vi "Main.vi"() -> ()   [LabVIEW 2015, in "Serializer.lvlib"]
doc: "This template is based from the Queued Message Handler design pattern and the Queued Message Handler Project Template that ships with LabVIEW 2014.\n\nThe main difference is that the Queue is private to this module and communication between modules is done via Broadcast and Requests events.\n\nRequests events are wrapped via public API methods and are handled in the Event handler loop in this VI.\nAny module can register for Broadcast events sent by this module.\n\nThe Event Handling Loop generates messages based on user interface actions.\n\nThe Message Handling Loop processes messages generated by the Event Handling Loop, or by other messages. The messages are string values, so new messages can be added easily to the Message Cases case structure in the Message Handling Loop. Each message cluster can also provide an optional value for Message Data, which is a variant that can be converted to whatever message-specific data is required.\n_____\nBased on Delacor QMH Project Template 3.1.0.34."
uses:
  Serializer.lvlib
  <vilib>/Delacor/Delacor QMH/Libraries/Cloneable Module Admin_class/Delacor_lib_QMH_Cloneable Module Admin.lvclass
  Module Data--cluster.ctl
  OOP/Serial/Base/Serial.lvclass
  <vilib>/Delacor/Delacor QMH/Libraries/Cloneable Module Admin_class/Delacor_lib_QMH_Cloneable Module Admin.lvclass/Delacor_lib_QMH_Cloneable Module Admin.ctl
  Stop Argument--cluster.ctl
  <vilib>/Delacor/Delacor QMH/Libraries/Module Admin_class/Delacor_lib_QMH_Module Admin.lvclass/Delacor_lib_QMH_Module Admin.ctl
  Send Argument--cluster.ctl
  config Argument--cluster.ctl
  Open Argument--cluster.ctl
  close Argument--cluster.ctl
  PollRX Argument--cluster.ctl
  <vilib>/Utility/miscctls.llb/LVPointTypeDef.ctl
  <vilib>/Delacor/Delacor QMH/Libraries/Cloneable Module Admin_class/Delacor_lib_QMH_Get Module ID.vi
  <vilib>/Delacor/Delacor QMH/Libraries/Module Admin_class/Delacor_lib_QMH_Get External Launch.vi
  <vilib>/Delacor/Delacor QMH/Libraries/Message Queue_class/Delacor_lib_QMH_Enqueue Message (Single).vi
  <vilib>/Utility/error.llb/Error Cluster From Error Code.vi
  <vilib>/ErrorRing/Error Ring.xnode
  <vilib>/Delacor/Delacor QMH/Libraries/Message Queue_class/Delacor_lib_QMH_Message Queue.lvclass
  Clone Registration/Clone Registration.lvlib
panel:
  in  "Simulate MHL Error":bool
  in  "Simulate EHL Error":bool
  out "error out":errorcluster
  in  "Module Admin":refnum<class "Delacor_lib_QMH_Cloneable Module Admin.lvclass">
  out "Status":string
  # "Other QMH Modules communicate with this Module via its Public API (wrappers for its Request Events).\n\nThis Module communicates with other Modules via its Broadcast Events.\nAny module that wants to get these messages, just registers for this module's Broadcast events."
  # "This template is for the Delacor Modified Queued Message Handler design pattern.\n\nSee the block diagram for more information on how to use this template."
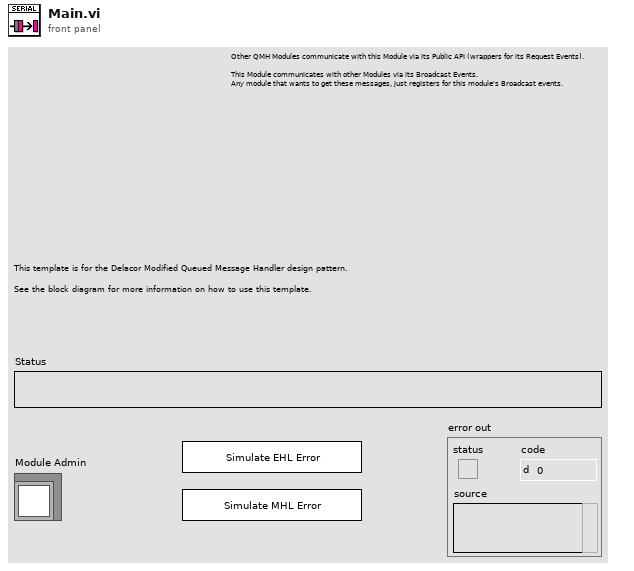
[diagram p1: front panel]
types:
  T1 = typedef "Serializer.lvlib/Request Events--cluster.ctl" = cluster{"Stop Module":refnum<user-event>, "Show Panel":refnum<user-event>, "Hide Panel":refnum<user-event>, "Show Diagram":refnum<user-event>, "Get Module Execution Status":refnum<user-event>, "Send":refnum<user-event>, "config":refnum<user-event>, "Open":refnum<user-event>, "close":refnum<user-event>, "PollRX":refnum<user-event>}
  T2 = typedef "Serializer.lvlib/Module Data--cluster.ctl" = cluster{"Status":string, "Serial.lvclass":refnum<class "Serial.lvclass">}
  T3 = typedef "Serializer.lvlib/Stop Argument--cluster.ctl" = cluster{"Origin":string, "Module ID":i32, "Exit via Stop Module Req?":bool, "Wait for Module to stop?":bool}
  T4 = typedef "Serializer.lvlib/Send Argument--cluster.ctl" = cluster{"Module ID":i32, "Bytes":u8[]}
  T5 = typedef "Serializer.lvlib/config Argument--cluster.ctl" = cluster{"Module ID":i32, "config":string}
  T6 = typedef "Serializer.lvlib/Open Argument--cluster.ctl" = cluster{"Module ID":i32, "Boolean":bool}
  T7 = typedef "Serializer.lvlib/close Argument--cluster.ctl" = cluster{"Module ID":i32, "Boolean":bool}
  T8 = typedef "Serializer.lvlib/PollRX Argument--cluster.ctl" = cluster{"Module ID":i32, "Boolean":bool}
  T9 = typedef "LVPointTypeDef.ctl" = cluster{"Horizontal":i16, "Vertical":i16}
  T10 = enum32{"Invalid", "Standard", "Closed", "Hidden", "Minimized", "Maximized"}
  T11 = enum32{"invalid lock state", "Not Locked", "Locked (No Password)", "Password-protected"}
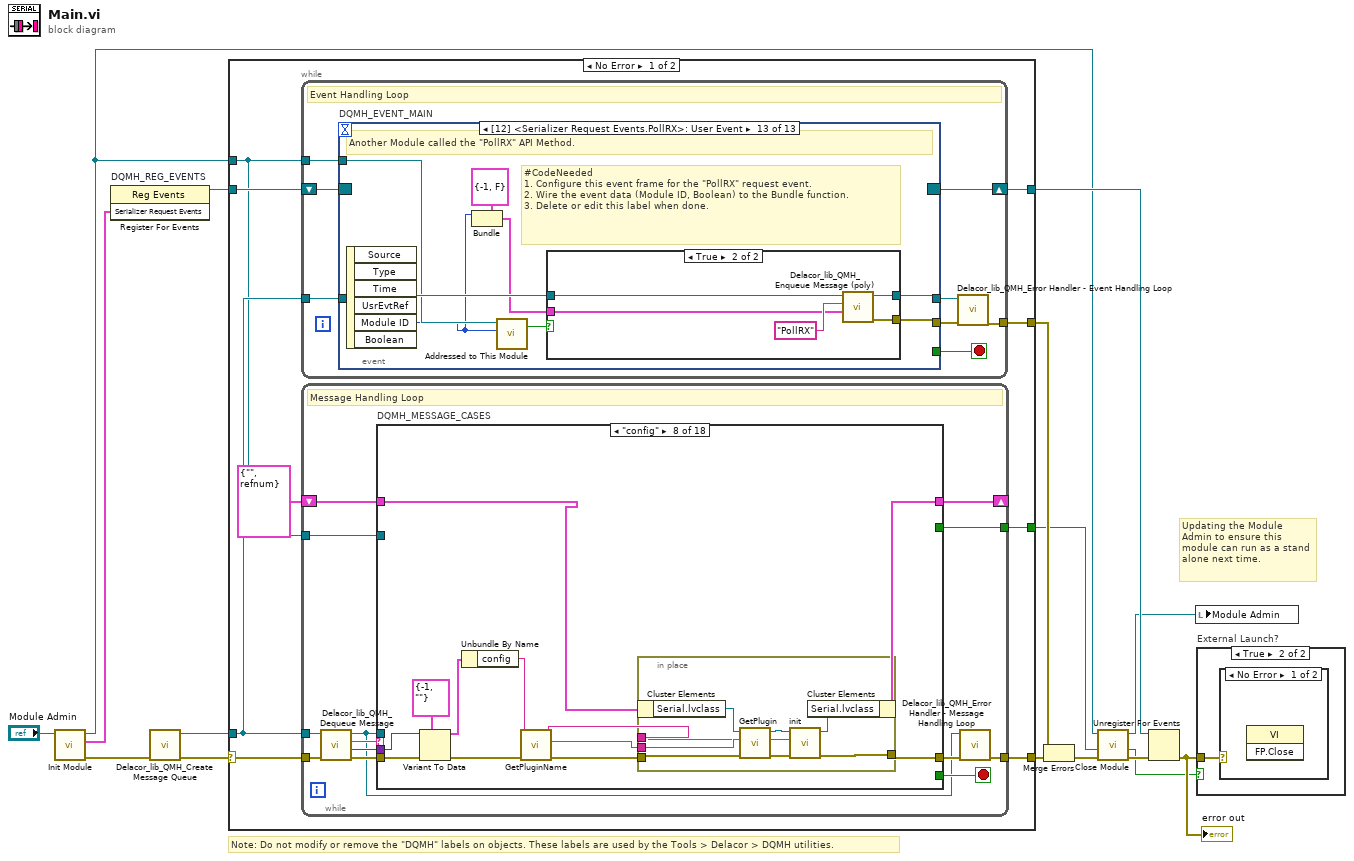
[diagram p0: block diagram]
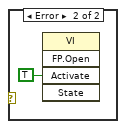
[diagram p3: hidden frame]
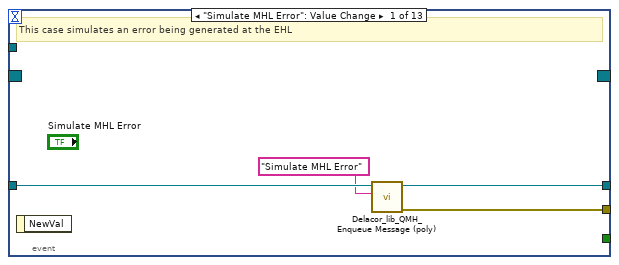
[diagram p4: hidden frame]
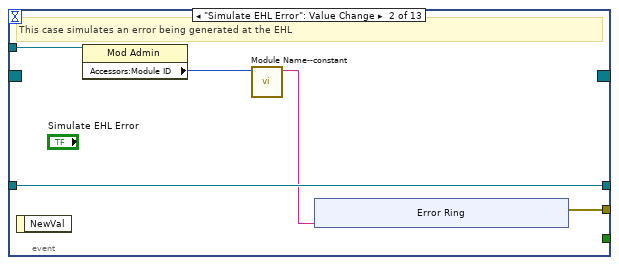
[diagram p5: hidden frame]
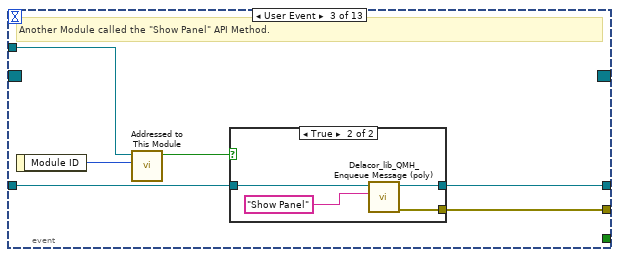
[diagram p6: hidden frame]
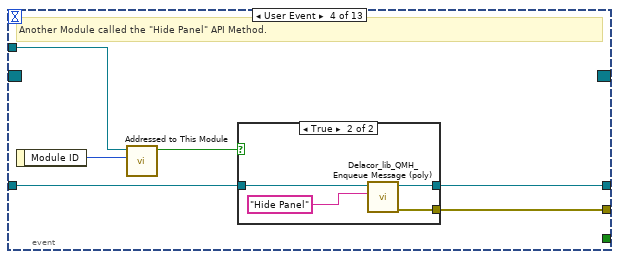
[diagram p8: hidden frame]
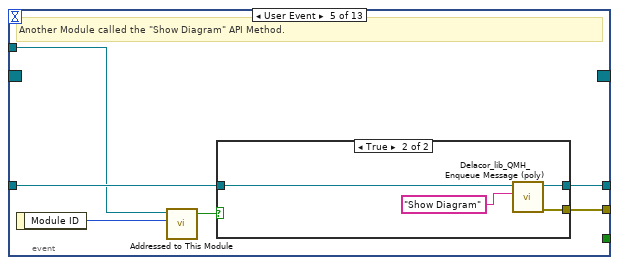
[diagram p10: hidden frame]
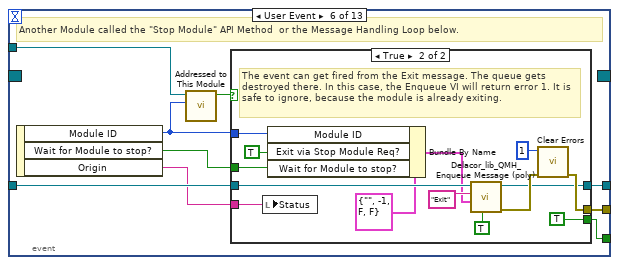
[diagram p12: hidden frame]
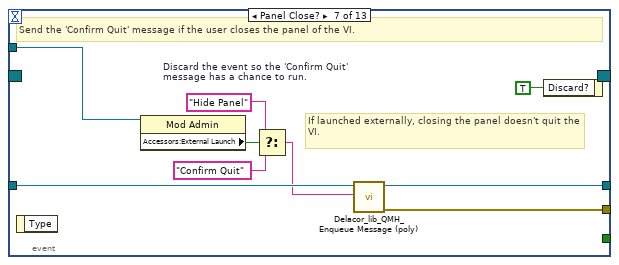
[diagram p14: hidden frame]
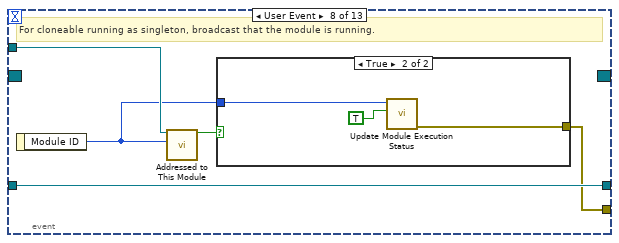
[diagram p15: hidden frame]
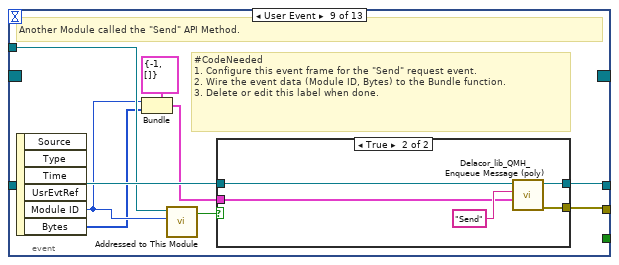
[diagram p17: hidden frame]
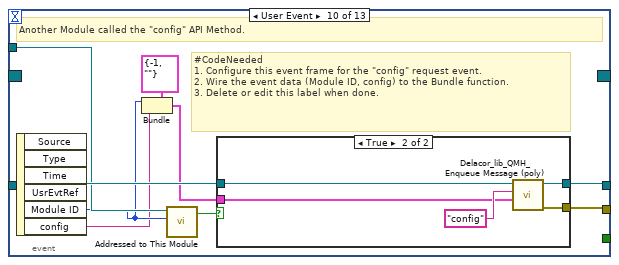
[diagram p19: hidden frame]
diagram:
  # "Note: Do not modify or remove the \"DQMH\" labels on objects. These labels are used by the Tools > Delacor > DQMH utilities."
  # "Updating the Module Admin to ensure this module can run as a stand alone next time."
  n1 = call "Init Module.vi"("Cloneable Module Admin in"="Module Admin") -> ("error out"=w13:errorcluster, "Serializer Request Events"=w10:T1, "Cloneable Module Admin out"=w6:refnum<class "Delacor_lib_QMH_Cloneable Module Admin.lvclass">)  [unwired: 8 in]
  n2 = register-events "DQMH_REG_EVENTS"(w10) -> (reference out=w11:refnum<event-registration>)  [unwired: 2 in, 1 out]
  n3 = call <vilib>:"Delacor_lib_QMH_Create Message Queue.vi"("error in (no error)"=w13) -> ("error out"=w1:errorcluster, "Message Queue out"=w9:refnum<class "Delacor_lib_QMH_Message Queue.lvclass">)  [unwired: 9 in]
  n4 = case shown="No Error" w1 {
    selector: w1 -> [w19 w447]
    tunnel: [w25 w447] -> w14
    tunnel: [w24 w448] -> w12
    tunnel: w11 -> [w22 w448]
    tunnel: w9 -> [w21 _]
    tunnel: [w20 _] -> w15
    tunnel: w6 -> [w18 w443]
    tunnel: [w17 _] -> w4
    frame No Error {
      n5 = while {
        tunnel: w21 -> [w33]
        shift-right: [w31] -> w24
        shift-left: w22 -> [w32]
        tunnel: [w27] -> w20
        tunnel: w18 -> [w26]
        stop <- w29 stop-if-true
        # "Event Handling Loop"
        n6 = event "DQMH_EVENT_MAIN" shown="[12] <Serializer Request Events.PollRX>: User Event" {
          selector: w32 -> [_ _ _ _ _ _ _ _ _ _ _ _ _]
          dyn-events: [_ _ _ _ _ _ _ _ _ _ _ _ _] -> w31
          timeout: _ -> [_ _ _ _ _ _ _ _ _ _ _ _ _]
          tunnel: [_ _ _ _ _ w86 _ _ _ _ _ _ _] -> w29
          tunnel: w33 -> [w37 w42 w55 w66 w77 w89 w114 w118 w132 w147 w161 w175 w189]
          tunnel: [w35 w41 w53 w64 w73 w91 w113 w117 w126 w141 w155 w169 w183] -> w30
          tunnel: [w36 w42 w54 w65 w76 w90 w112 w118 w131 w146 w160 w174 w188] -> w28
          tunnel: w26 -> [_ w40 w50 w61 w74 w88 w108 w119 w129 w144 w158 w172 w186]
          event "Simulate MHL Error": Value Change {
            # "This case simulates an error being generated at the EHL"
            n7 = event-data() -> ()  [unwired: 1 in, 1 out]
            n8 = call-poly <vilib>:"Delacor_lib_QMH_Enqueue Message (poly).vi"("Message"="Simulate MHL Error", "Message Queue in"=w37) -> ("error out"=w35:errorcluster, "Message Queue out"=w36:refnum<class "Delacor_lib_QMH_Message Queue.lvclass">)  [unwired: 8 in]
          }
          event "Simulate EHL Error": Value Change {
            # "This case simulates an error being generated at the EHL"
            n9 = event-data() -> ()  [unwired: 1 in, 1 out]
            n10 = property class="Mod Admin"(reference=w40) -> ("Accessors:Module ID"=w39:i32)  [unwired: 1 in, 2 out]
            n11 = call "Module Name--constant.vi"("Module ID"=w39) -> ("Module Name"=w38:string)  [unwired: 10 in]
            n12 = xnode "Error Ring"("parameter 0"=w38) -> ("error out"=w41:errorcluster)
          }
          event User Event {
            # "Another Module called the \"Show Panel\" API Method."
            n13 = event-data() -> ("Module ID"=w52:i32)  [unwired: 1 in]
            n14 = call "Addressed to This Module.vi"("Module ID from Argument"=w52, "Module Admin"=w50) -> ("Addressed to this instance?"=w51:bool)  [unwired: 8 in, 1 out]
            n15 = case shown="True" w51 {
              tunnel: w55 -> [w56 w60]
              tunnel: [w56 w59] -> w54
              tunnel: [_ w58] -> w53
              frame False {
              }
              frame True {
                n16 = call-poly <vilib>:"Delacor_lib_QMH_Enqueue Message (poly).vi"("Message"="Show Panel", "Message Queue in"=w60) -> ("error out"=w58:errorcluster, "Message Queue out"=w59:refnum<class "Delacor_lib_QMH_Message Queue.lvclass">)  [unwired: 8 in]
              }
            }
          }
          event User Event {
            # "Another Module called the \"Hide Panel\" API Method."
            n17 = event-data() -> ("Module ID"=w63:i32)  [unwired: 1 in]
            n18 = call "Addressed to This Module.vi"("Module ID from Argument"=w63, "Module Admin"=w61) -> ("Addressed to this instance?"=w62:bool)  [unwired: 8 in, 1 out]
            n19 = case shown="True" w62 {
              tunnel: w66 -> [w67 w71]
              tunnel: [w67 w70] -> w65
              tunnel: [_ w69] -> w64
              frame False {
              }
              frame True {
                n20 = call-poly <vilib>:"Delacor_lib_QMH_Enqueue Message (poly).vi"("Message"="Hide Panel", "Message Queue in"=w71) -> ("error out"=w69:errorcluster, "Message Queue out"=w70:refnum<class "Delacor_lib_QMH_Message Queue.lvclass">)  [unwired: 8 in]
              }
            }
          }
          event User Event {
            # "Another Module called the \"Show Diagram\" API Method."
            n21 = event-data() -> ("Module ID"=w72:i32)  [unwired: 1 in]
            n22 = call "Addressed to This Module.vi"("Module ID from Argument"=w72, "Module Admin"=w74) -> ("Addressed to this instance?"=w75:bool)  [unwired: 8 in, 1 out]
            n23 = case shown="True" w75 {
              tunnel: w77 -> [w78 w82]
              tunnel: [w78 w81] -> w76
              tunnel: [_ w79] -> w73
              frame False {
              }
              frame True {
                n24 = call-poly <vilib>:"Delacor_lib_QMH_Enqueue Message (poly).vi"("Message"="Show Diagram", "Message Queue in"=w82) -> ("error out"=w79:errorcluster, "Message Queue out"=w81:refnum<class "Delacor_lib_QMH_Message Queue.lvclass">)  [unwired: 8 in]
              }
            }
          }
          event User Event {
            # "Another Module called the \"Stop Module\" API Method  or the Message Handling Loop below."
            n25 = event-data() -> ("Module ID"=w84:i32, "Wait for Module to stop?"=w85:bool, "Origin"=w83:string)  [unwired: 1 in]
            n26 = call "Addressed to This Module.vi"("Module ID from Argument"=w84, "Module Admin"=w88) -> ("Addressed to this instance?"=w87:bool)  [unwired: 8 in, 1 out]
            n27 = case shown="True" w87 {
              tunnel: [_ w102] -> w91
              tunnel: [w92 w101] -> w90
              tunnel: w89 -> [w92 w100]
              tunnel: [_ TRUE] -> w86
              tunnel: w85 -> [_ w95]
              tunnel: w84 -> [_ w97]
              tunnel: w83 -> [_ w93]
              frame False {
              }
              frame True {
                # "The event can get fired from the Exit message. The queue gets destroyed there. In this case, the Enqueue VI will return error 1. It is safe to ignore, because the module is already exiting."
                n28 = local write "Status"(w93) -> ()
                n29 = Bundle By Name(cluster=T3 {"Origin"="", "Module ID"=-1, "Exit via Stop Module Req?"=FALSE, "Wait for Module to stop?"=FALSE} ("Stop Argument"), "Module ID"=w97, "Exit via Stop Module Req?"=TRUE, "Wait for Module to stop?"=w95) -> (w94:T3)
                n30 = call-poly <vilib>:"Delacor_lib_QMH_Enqueue Message (poly).vi"("Priority Message? (F)"=TRUE, "Message Data"=w94, "Message"="Exit", "Message Queue in"=w100) -> ("error out"=w105:errorcluster, "Message Queue out"=w101:refnum<class "Delacor_lib_QMH_Message Queue.lvclass">)  [unwired: 6 in]
                n31 = call <vilib>:"Clear Errors.vi"("error in (no error)"=w105, "specific error code to clear (0: all)"=1) -> ("error out"=w102:errorcluster)  [unwired: 4 in, 1 out]
              }
            }
          }
          event Panel Close? {
            w115 = TRUE  # Discard the event so the 'Confirm Quit' message has a chance to run.
            # "If launched externally, closing the panel doesn't quit the VI."
            # "Send the 'Confirm Quit' message if the user closes the panel of the VI."
            n32 = event-data() -> ()  [unwired: 1 in, 1 out]
            n33 = property class="Mod Admin"(reference=w108) -> ("Accessors:External Launch"=w107:bool)  [unwired: 1 in, 2 out]
            n34 = Select(t="Hide Panel" ("Message"), s=w107, f="Confirm Quit" ("Message")) -> (s? t:f=w109:string)
            n35 = call-poly <vilib>:"Delacor_lib_QMH_Enqueue Message (poly).vi"("Message"=w109, "Message Queue in"=w114) -> ("error out"=w113:errorcluster, "Message Queue out"=w112:refnum<class "Delacor_lib_QMH_Message Queue.lvclass">)  [unwired: 8 in]
            n36 = event-data("Discard?"=w115) -> ()  [unwired: 1 in, 1 out]
          }
          event User Event {
            # "For cloneable running as singleton, broadcast that the module is running."
            n37 = event-data() -> ("Module ID"=w116:i32)  [unwired: 1 in]
            n38 = call "Addressed to This Module.vi"("Module ID from Argument"=w116, "Module Admin"=w119) -> ("Addressed to this instance?"=w120:bool)  [unwired: 8 in, 1 out]
            n39 = case shown="True" w120 {
              tunnel: [_ w123] -> w117
              tunnel: w116 -> [_ w122]
              frame False {
              }
              frame True {
                n40 = call "Update Module Execution Status.vi"("Running?"=TRUE, "Module ID"=w122) -> ("error out"=w123:errorcluster)  [unwired: 9 in]
              }
            }
          }
          event User Event {
            # "#CodeNeeded\n1. Configure this event frame for the \"Send\" request event.\n2. Wire the event data (Module ID, Bytes) to the Bundle function.\n3. Delete or edit this label when done."
            # "Another Module called the \"Send\" API Method."
            n41 = event-data() -> ("Module ID"=w125:i32, "Bytes"=w124:u8[])  [unwired: 1 in, 4 out]
            n42 = Bundle(cluster=T4 {"Module ID"=-1, "Bytes"=[]} ("Send Argument"), "Module ID"=w125, "Bytes"=w124) -> (w127:T4)
            n43 = call "Addressed to This Module.vi"("Module ID from Argument"=w125, "Module Admin"=w129) -> ("Addressed to this instance?"=w130:bool)  [unwired: 8 in, 1 out]
            n44 = case shown="True" w130 {
              tunnel: w132 -> [w133 w138]
              tunnel: [w133 w137] -> w131
              tunnel: w127 -> [_ w135]
              tunnel: [_ w134] -> w126
              frame False {
              }
              frame True {
                n45 = call-poly <vilib>:"Delacor_lib_QMH_Enqueue Message (poly).vi"("Message Data"=w135, "Message"="Send", "Message Queue in"=w138) -> ("error out"=w134:errorcluster, "Message Queue out"=w137:refnum<class "Delacor_lib_QMH_Message Queue.lvclass">)  [unwired: 7 in]
              }
            }
          }
          event User Event {
            # "#CodeNeeded\n1. Configure this event frame for the \"config\" request event.\n2. Wire the event data (Module ID, config) to the Bundle function.\n3. Delete or edit this label when done."
            # "Another Module called the \"config\" API Method."
            n46 = event-data() -> ("Module ID"=w140:i32, "config"=w139:string)  [unwired: 1 in, 4 out]
            n47 = Bundle(cluster=T5 {"Module ID"=-1, "config"=""} ("config Argument"), "Module ID"=w140, "config"=w139) -> (w142:T5)
            n48 = call "Addressed to This Module.vi"("Module ID from Argument"=w140, "Module Admin"=w144) -> ("Addressed to this instance?"=w145:bool)  [unwired: 8 in, 1 out]
            n49 = case shown="True" w145 {
              tunnel: w147 -> [w148 w153]
              tunnel: [w148 w152] -> w146
              tunnel: w142 -> [_ w150]
              tunnel: [_ w149] -> w141
              frame False {
              }
              frame True {
                n50 = call-poly <vilib>:"Delacor_lib_QMH_Enqueue Message (poly).vi"("Message Data"=w150, "Message"="config", "Message Queue in"=w153) -> ("error out"=w149:errorcluster, "Message Queue out"=w152:refnum<class "Delacor_lib_QMH_Message Queue.lvclass">)  [unwired: 7 in]
              }
            }
          }
          event User Event {
            # "#CodeNeeded\n1. Configure this event frame for the \"Open\" request event.\n2. Wire the event data (Module ID, Boolean) to the Bundle function.\n3. Delete or edit this label when done."
            # "Another Module called the \"Open\" API Method."
            n51 = event-data() -> ("Module ID"=w154:i32)  [unwired: 1 in, 5 out]
            n52 = Bundle(cluster=T6 {"Module ID"=-1, "Boolean"=FALSE} ("Open Argument"), "Module ID"=w154) -> (w156:T6)  [unwired: 1 in]
            n53 = call "Addressed to This Module.vi"("Module ID from Argument"=w154, "Module Admin"=w158) -> ("Addressed to this instance?"=w159:bool)  [unwired: 8 in, 1 out]
            n54 = case shown="True" w159 {
              tunnel: w161 -> [w162 w167]
              tunnel: [w162 w166] -> w160
              tunnel: w156 -> [_ w164]
              tunnel: [_ w163] -> w155
              frame False {
              }
              frame True {
                n55 = call-poly <vilib>:"Delacor_lib_QMH_Enqueue Message (poly).vi"("Message Data"=w164, "Message"="Open", "Message Queue in"=w167) -> ("error out"=w163:errorcluster, "Message Queue out"=w166:refnum<class "Delacor_lib_QMH_Message Queue.lvclass">)  [unwired: 7 in]
              }
            }
          }
          event User Event {
            # "#CodeNeeded\n1. Configure this event frame for the \"close\" request event.\n2. Wire the event data (Module ID, Boolean) to the Bundle function.\n3. Delete or edit this label when done."
            # "Another Module called the \"close\" API Method."
            n56 = event-data() -> ("Module ID"=w168:i32)  [unwired: 1 in, 5 out]
            n57 = Bundle(cluster=T7 {"Module ID"=-1, "Boolean"=FALSE} ("close Argument"), "Module ID"=w168) -> (w170:T7)  [unwired: 1 in]
            n58 = call "Addressed to This Module.vi"("Module ID from Argument"=w168, "Module Admin"=w172) -> ("Addressed to this instance?"=w173:bool)  [unwired: 8 in, 1 out]
            n59 = case shown="True" w173 {
              tunnel: w175 -> [w176 w181]
              tunnel: [w176 w180] -> w174
              tunnel: w170 -> [_ w178]
              tunnel: [_ w177] -> w169
              frame False {
              }
              frame True {
                n60 = call-poly <vilib>:"Delacor_lib_QMH_Enqueue Message (poly).vi"("Message Data"=w178, "Message"="close", "Message Queue in"=w181) -> ("error out"=w177:errorcluster, "Message Queue out"=w180:refnum<class "Delacor_lib_QMH_Message Queue.lvclass">)  [unwired: 7 in]
              }
            }
          }
          event User Event {
            # "#CodeNeeded\n1. Configure this event frame for the \"PollRX\" request event.\n2. Wire the event data (Module ID, Boolean) to the Bundle function.\n3. Delete or edit this label when done."
            # "Another Module called the \"PollRX\" API Method."
            n61 = event-data() -> ("Module ID"=w182:i32)  [unwired: 1 in, 5 out]
            n62 = Bundle(cluster=T8 {"Module ID"=-1, "Boolean"=FALSE} ("PollRX Argument"), "Module ID"=w182) -> (w184:T8)  [unwired: 1 in]
            n63 = call "Addressed to This Module.vi"("Module ID from Argument"=w182, "Module Admin"=w186) -> ("Addressed to this instance?"=w187:bool)  [unwired: 8 in, 1 out]
            n64 = case shown="True" w187 {
              tunnel: w189 -> [w190 w195]
              tunnel: [w190 w194] -> w188
              tunnel: w184 -> [_ w192]
              tunnel: [_ w191] -> w183
              frame False {
              }
              frame True {
                n65 = call-poly <vilib>:"Delacor_lib_QMH_Enqueue Message (poly).vi"("Message Data"=w192, "Message"="PollRX", "Message Queue in"=w195) -> ("error out"=w191:errorcluster, "Message Queue out"=w194:refnum<class "Delacor_lib_QMH_Message Queue.lvclass">)  [unwired: 7 in]
              }
            }
          }
        }
        n66 = call-dynamic "Delacor_lib_QMH_Error Handler - Event Handling Loop.vi"("error in (no error)"=w30, "Message Queue in"=w28) -> ("dup error in"=w27:errorcluster)  [unwired: 8 in, 1 out]
      }
      n67 = while {
        tunnel: w21 -> [w200]
        shift-right: [w206] -> _
        shift-left: T2 {"Status"="", "Serial.lvclass"=refnum} ("Data Cluster") -> [w207]
        tunnel: w19 -> [w204]
        tunnel: [w198] -> w25
        tunnel: w18 -> [w197]
        tunnel: [w196] -> w17
        stop <- w205 stop-if-true
        # "Message Handling Loop"
        n68 = call-dynamic "Delacor_lib_QMH_Dequeue Message.vi"("error in (no error)"=w204, "Message Queue in"=w200) -> ("error out"=w203:errorcluster, "Message Data"=w201:variant, "Message"=w202:string, "Message Queue out"=w199:refnum<class "Delacor_lib_QMH_Message Queue.lvclass">)  [unwired: 6 in]
        n69 = case "DQMH_MESSAGE_CASES" shown="\"config\"" w202 {
          selector: w202 -> [_ _ _ _ _ _ _ _ _ _ _ _ _ _ _ _ _ w430]
          tunnel: w199 -> [_ _ _ _ _ _ _ _ _ _ _ _ _ w374 _ w407 w424 _]
          tunnel: w203 -> [w221 w237 w245 w251 w254 w275 w286 w298 w315 w328 w346 w369 w372 w383 w396 w406 w426 _]
          tunnel: [w214 w238 w245 w251 w253 w273 w276 w293 w310 w322 w337 w367 w370 w373 w394 w405 w420 w431] -> w208
          tunnel: w207 -> [w220 w239 w244 w250 w255 w274 w281 w288 w309 w325 w342 w368 w371 w382 w395 w410 w423 w432]
          tunnel: [w219 w239 w244 w250 w255 w274 w280 w294 w308 w324 w341 w368 w371 w382 w395 w410 w423 w432] -> w206
          tunnel: [_ _ _ _ _ _ _ _ _ _ _ _ _ _ _ _ w422 _] -> w205
          tunnel: w201 -> [_ w236 _ _ _ _ w285 w297 w314 w327 w345 _ _ w381 _ _ w416 _]
          tunnel: w197 -> [w211 w231 w242 w249 w252 _ _ _ _ _ _ _ _ w378 w391 _ w412 w428]
          tunnel: [_ _ _ _ _ _ _ _ _ _ _ _ _ _ _ _ w414 _] -> w196
          frame "Initialize" {
            w218 = "Initial Message" ("Initial Message")
            # "#CodeNeeded - Initialize the appearance of the front panel."
            # "#CodeNeeded - Initialize your state data here."
            # "Initialize - Any operation that needs to be done before the module can receive messages. Synchronize Caller Events.vi will inform Start Module.vi that the module has launched and is ready to receive messages. Module Did Init.vi will broadcast that the module initialized."
            n70 = call "Synchronize Caller Events.vi"("error in (no error)"=w221, "Module Admin"=w211) -> ("error out"=w215:errorcluster, "Module Admin out"=w210:refnum<class "Delacor_lib_QMH_Cloneable Module Admin.lvclass">)  [unwired: 8 in]
            n71 = property class="Mod Admin"(reference=w210) -> ("Accessors:Module ID"=w213:i32, "Accessors:External Launch"=w212:bool)  [unwired: 1 in, 2 out]
            n72 = call "Module Name--constant.vi"("Module ID"=w213) -> ("Module Name"=w225:string)  [unwired: 10 in]
            n73 = property class="VI"("Front Panel.Title"=w225) -> (reference out=w228:refnum<vi>, error out=w229:errorcluster)  [unwired: 2 in]
            n74 = Select(t=T10."Hidden" ("State"), s=w212, f=T10."Standard" ("State")) -> (s? t:f=w222:T10)
            n75 = invoke class="VI" method="FP.Open"(reference=w228, error in=w229, "State"=w222) -> (reference out=w227:refnum<vi>, error out=w226:errorcluster)  [unwired: 2 in, 3 out]
            n76 = call "Module Name--constant.vi"("Module ID"=w213) -> ("Module Name"=w216:string)  [unwired: 10 in]
            n77 = Bundle By Name(cluster=w220, "Status"=w218) -> (w219:T2)
            n78 = local write "Status"(w218) -> ()
            n79 = invoke class="VI" method="FP.Center"(reference=w227, error in=w226) -> ()  [unwired: 1 in, 3 out]
            n80 = property on="Pane" class="Pane"("Origin"=T9 {"Horizontal"=0, "Vertical"=0}) -> ()  [unwired: 2 in, 2 out]
            n81 = call "Module Did Init.vi"("error in (no error)"=w215, "Initialized?"=TRUE, "Origin"=w216, "Module ID"=w213) -> ("error out"=w214:errorcluster)  [unwired: 7 in]
          }
          frame "Update Display" {
            # "Broadcast updated status to any VI registered to listen to this module's broadcast events."
            # "Convert the message data to a string to display in the Status indicator."
            # "#CodeRecommended - If you wish to decouple the Message Handling Loop from your user interface, consider creating User Events (like the \"Stop\" event in this VI) to message the Event Handling Loop whenever the user interface needs updating."
            # "Update Display - Update user interface here."
            n82 = Variant To Data(error in=w237, type="", Variant=w236) -> (data=w234:string, error out=w233:errorcluster)
            "Status" <- w234
            n83 = property class="Mod Admin"(reference=w231) -> ("Accessors:Module ID"=w230:i32)  [unwired: 1 in, 2 out]
            n84 = call "Status Updated.vi"("error in (no error)"=w233, "Status"=w234, "Module ID"=w230) -> ("error out"=w232:errorcluster)  [unwired: 8 in]
            n85 = Merge Errors(w232) -> (w238:errorcluster)
          }
          frame "Show Panel" {
            # "Show the panel of this VI, and send a status updated message to let listeners know."
            n86 = property class="Mod Admin"(reference=w242) -> ("Accessors:Module ID"=w241:i32)  [unwired: 1 in, 2 out]
            n87 = call "Status Updated.vi"("Status"="Panel shown." ("format string"), "Module ID"=w241) -> ()  [unwired: 9 in, 1 out]
            n88 = invoke class="VI" method="FP.Open"("Activate"=TRUE ("Activate?")) -> ()  [unwired: 4 in, 5 out]
          }
          frame "Hide Panel" {
            # "Hide the panel of this VI, and send a status updated message to let listeners know."
            n89 = property class="Mod Admin"(reference=w249) -> ("Accessors:Module ID"=w248:i32)  [unwired: 1 in, 2 out]
            n90 = call "Status Updated.vi"("Status"="Panel hidden." ("format string"), "Module ID"=w248) -> ()  [unwired: 9 in, 1 out]
            n91 = invoke class="VI" method="FP.Open"("State"=T10."Hidden") -> ()  [unwired: 4 in, 5 out]
          }
          frame "Show Diagram" {
            # "Show Diagram - Show the block diagram of this VI. Used as a debugging tool. There is a button in the module tester that fires the Show Diagram request, which runs this message. Note that the diagram will not be displayed if it is password-protected and the password is not in the cache."
            n92 = disable-structure shown="RUN_TIME_ENGINE==False" {
              disable-tunnel: [w264 w272] -> w253
              disable-tunnel: w254 -> [w263 w272]
              disable-tunnel: w252 -> [w256 _]
              frame condition #0 (active) {
                # "functionality not available in exe"
                n93 = invoke class="VI" method="Lock State.Get"(error in=w263) -> (error out=w262:errorcluster, "Get Lock State"=w261:T11, "pwd in cache"=w258:bool)  [unwired: 3 in, 1 out]
                n94 = Equal?(x=T11."Password-protected", y=w261) -> (x = y?=w259:bool)
                n95 = Compound Arithmetic op=AND(w259, invert w258) -> (w257:bool)
                n96 = case shown="False" w257 {
                  tunnel: [w269 w271] -> w264
                  tunnel: w262 -> [w268 w271]
                  tunnel: w256 -> [w265 _]
                  frame False {
                    n97 = property class="Mod Admin"(reference=w265) -> ("Accessors:Module ID"=w266:i32)  [unwired: 1 in, 2 out]
                    n98 = property class="VI"(error in=w268, "BDWin.Open"=TRUE ("Block Diagram Window:Open")) -> (error out=w269:errorcluster)  [unwired: 1 in, 1 out]
                    n99 = call "Status Updated.vi"("Status"="Block Diagram shown." ("format string"), "Module ID"=w266) -> ()  [unwired: 9 in, 1 out]
                  }
                  frame True {
                    # "Password-protected VI, and the password is not in the cache. Do not show the diagram."
                  }
                }
              }
              frame condition #1 {
              }
            }
          }
          frame "--- Module Specific ---" {
            # "Separator -- The following cases handle messages specific to this Module."
            n100 = Merge Errors(w275) -> (w273:errorcluster)
          }
          frame "Send" {
            n101 = Variant To Data(error in=w286, type=T4 {"Module ID"=-1, "Bytes"=[]} ("Send Argument"), Variant=w285) -> (data=w283:T4, error out=w277:errorcluster)
            n102 = Unbundle By Name(w283) -> ("Bytes"=w278:u8[])  [unwired: 1 out]
            n103 = Unbundle By Name(w281) -> ("Serial.lvclass"=w282:refnum<class "Serial.lvclass">)
            n104 = call-dynamic "send.vi"("error in (no error)"=w277, "Bytes"=w278, "Serial in"=w282) -> ("error out"=w276:errorcluster, "Serial out"=w279:refnum<class "Serial.lvclass">)  [unwired: 7 in]
            n105 = Bundle By Name(cluster=w281, "Serial.lvclass"=w279) -> (w280:T2)
          }
          frame "config" {
            n106 = Variant To Data(error in=w298, type=T5 {"Module ID"=-1, "config"=""} ("config Argument"), Variant=w297) -> (data=w295:T5, error out=w291:errorcluster)
            n107 = Unbundle By Name(w295) -> ("config"=w292:string)
            n108 = call "GetPluginName.vi"("error in (no error)"=w291, "config"=w292) -> ("error out"=w289:errorcluster, "Plugin"=w287:string, "config(out)"=w290:string)  [unwired: 7 in]
            n109 = in-place {
              in-place-border: w290 -> [w300]
              in-place-border: w289 -> [w301]
              in-place-border: [w305] -> w293
              in-place-border: w287 -> [w302]
              n110 = in-place-cluster #1(w288) -> ("Serial.lvclass"=w304:refnum<class "Serial.lvclass">)
              n111 = call "GetPlugin.vi"("error in (no error)"=w301, "name or relative path"=w302, "Serializer.lvlib:Serial.lvclass"=w304) -> ("error out"=w299:errorcluster, "serialClass"=w303:refnum<class "Serial.lvclass">)  [unwired: 7 in]
              n112 = call-dynamic "init.vi"("error in (no error)"=w299, "Config"=w300, "Serial in"=w303) -> ("error out"=w305:errorcluster, "Serial out"=w306:refnum<class "Serial.lvclass">)  [unwired: 7 in]
              n113 = in-place-cluster #1("Serial.lvclass"=w306) -> (w294:T2)
            }
          }
          frame "Open" {
            n114 = Variant To Data(error in=w315, type=T6 {"Module ID"=-1, "Boolean"=FALSE} ("Open Argument"), Variant=w314) -> (data=w312:T6, error out=w311:errorcluster)
            n115 = Unbundle By Name(w312) -> ("Module ID"=w307:i32)  [unwired: 1 out]
            n116 = in-place {
              in-place-border: w311 -> [w319]
              in-place-border: [w317] -> w310
              in-place-border: w307 -> [w316]
              n117 = in-place-cluster #2(w309) -> ("Serial.lvclass"=w321:refnum<class "Serial.lvclass">)
              n118 = call-dynamic "open.vi"("error in (no error)"=w319, "Serial in"=w321) -> ("error out"=w318:errorcluster, "Serial out"=w320:refnum<class "Serial.lvclass">)  [unwired: 8 in]
              n119 = call "PollRX.vi"("error in (no error)"=w318, "Module ID"=w316) -> ("error out"=w317:errorcluster)  [unwired: 9 in]
              n120 = in-place-cluster #2("Serial.lvclass"=w320) -> (w308:T2)
            }
          }
          frame "close" {
            n121 = Variant To Data(error in=w328, type=T7 {"Module ID"=-1, "Boolean"=FALSE} ("close Argument"), Variant=w327) -> (error out=w323:errorcluster)  [unwired: 1 out]
            n122 = in-place {
              in-place-border: w323 -> [w330]
              in-place-border: [w329] -> w322
              n123 = in-place-cluster #3(w325) -> ("Serial.lvclass"=w332:refnum<class "Serial.lvclass">)
              n124 = call-dynamic "close.vi"("error in (no error)"=w330, "Serial in"=w332) -> ("error out"=w329:errorcluster, "Serial out"=w331:refnum<class "Serial.lvclass">)  [unwired: 8 in]
              n125 = in-place-cluster #3("Serial.lvclass"=w331) -> (w324:T2)
            }
          }
          frame "PollRX" {
            n126 = Variant To Data(error in=w346, type=T8 {"Module ID"=-1, "Boolean"=FALSE} ("PollRX Argument"), Variant=w345) -> (data=w339:T8, error out=w343:errorcluster)
            n127 = in-place {
              in-place-border: w343 -> [w365]
              in-place-border: [w364] -> w335
              in-place-border: [w362] -> w340
              n128 = in-place-cluster #4(w342) -> ("Serial.lvclass"=w366:refnum<class "Serial.lvclass">)
              n129 = call-dynamic "read.vi"("error in (no error)"=w365, "Serial in"=w366) -> ("error out"=w364:errorcluster, "Bytes"=w362:u8[], "Serial out"=w363:refnum<class "Serial.lvclass">)  [unwired: 7 in]
              n130 = in-place-cluster #4("Serial.lvclass"=w363) -> (w341:T2)
            }
            n131 = Unbundle By Name(w339) -> ("Module ID"=w338:i32)
            n132 = call <vilib>:"Clear Errors.vi"("error in (no error)"=w335, "specific error code to clear (0: all)"=1) -> ("error out"=w336:errorcluster, "specific error cleared?"=w333:bool)  [unwired: 4 in]
            n133 = case shown="True" w333 {
              tunnel: w340 -> [w350 _]
              tunnel: w338 -> [w349 _]
              tunnel: [w348 w361] -> w337
              tunnel: w336 -> [w347 w361]
              frame False {
                n134 = Array Size(array=w350) -> (size(s)=w351:i32)
                n135 = case shown="Default" w351 {
                  tunnel: [w352 w358] -> w348
                  tunnel: w347 -> [w356 w359]
                  tunnel: w350 -> [w355 _]
                  tunnel: w349 -> [w354 w360]
                  frame Default {
                    n136 = call "Received.vi"("error in (no error)"=w356, "Bytes"=w355, "Module ID"=w354) -> ("error out"=w353:errorcluster)  [unwired: 8 in]
                    n137 = call "PollRX.vi"("error in (no error)"=w353, "Module ID"=w354) -> ("error out"=w352:errorcluster)  [unwired: 9 in]
                  }
                  frame 0 {
                    n138 = call "LaunchDelRx.vi"("error in (no error)"=w359, "milliseconds to wait"=u32 50, "Module ID"=w360) -> ("error out"=w358:errorcluster)  [unwired: 8 in]
                  }
                }
              }
              frame True {
              }
            }
          }
          frame "---Copy This Frame---" {
            # "Duplicate this frame when creating new messages.  Change this comment in the duplicated frame to describe this message."
            n139 = Merge Errors(w369) -> (w367:errorcluster)
          }
          frame "--- Exit and Error Handling---" {
            # "Separator - the following cases handle errors and exit messages."
            n140 = Merge Errors(w372) -> (w370:errorcluster)
          }
          frame "Error" {
            # "#CodeRecommended - If you ever change the name of this \"Error\" message, you'll need to update the name in the Check Loop Error.vi as well."
            # "#CodeRecommended - If the module is running in standalone mode (External Launch = FALSE), this code will pop up an error dialog and call the 'Exit' message if an error occurs. Add more fine-grained error handling here."
            # "Error - Check the error message data and respond accordingly. This message is sent by the \"Error Handler\" VIs at the end of each loop in this application."
            n141 = property class="Mod Admin"(reference=w378) -> ("Accessors:External Launch"=w375:bool, "Accessors:Module ID"=w377:i32)  [unwired: 1 in, 2 out]
            n142 = Variant To Data(error in=w383, type=errorcluster {"status"=FALSE, "code"=0, "source"=""} ("error constant"), Variant=w381) -> (data=w384:errorcluster, error out=w379:errorcluster)
            n143 = call "Error Reported.vi"("Error"=w384, "Module ID"=w377) -> ()  [unwired: 9 in, 1 out]
            n144 = case shown="False" w375 {
              tunnel: [w389 _] -> w376
              tunnel: w374 -> [w388 _]
              tunnel: w384 -> [w385 _]
              frame False {
                # "If the module is running standalone, then pop up an error dialog and call the \"Exit\" message."
                n145 = call <vilib>:"Simple Error Handler.vi"("error in (no error)"=w385) -> ()  [unwired: 4 in, 5 out]
                n146 = call-poly <vilib>:"Delacor_lib_QMH_Enqueue Message (poly).vi"("Priority Message? (F)"=TRUE, "Message"="Exit", "Message Queue in"=w388) -> ("error out"=w389:errorcluster)  [unwired: 7 in, 1 out]
              }
              frame True {
                # "If the module was launched externally, calling the Error Reported broadcast VI is the only action performed by the \"Error\" message. The module's caller can then process the error appropriately."
              }
            }
            n147 = Merge Errors(w379, w376) -> (w373:errorcluster)
            n148 = local write "error out"(w373) -> ()
          }
          frame "Simulate MHL Error" {
            # "Simulate an error occurring at the MHL"
            n149 = property class="Mod Admin"(reference=w391) -> ("Accessors:Module ID"=w392:i32)  [unwired: 1 in, 2 out]
            n150 = call "Module Name--constant.vi"("Module ID"=w392) -> ("Module Name"=w390:string)  [unwired: 10 in]
            n151 = xnode "Error Ring"("parameter 0"=w390) -> ("error out"=w393:errorcluster)
            n152 = Merge Errors(w396, w393) -> (w394:errorcluster)
          }
          frame "Confirm Quit" {
            # "#CodeNeeded - If you want to provide an \"Are you sure\" dialog (or some other notification) before the application exits, place that code here. This message is typically sent from a Panel Close? event."
            # "Confirm Quit - Message that can confirm whether or not the user wants to exit this instance."
            n153 = call-poly <vilib>:"Delacor_lib_QMH_Enqueue Message (poly).vi"("Priority Message? (F)"=TRUE, "error in (no error)"=w406, "Message"="Exit", "Message Queue in"=w407) -> ("error out"=w409:errorcluster)  [unwired: 6 in, 1 out]
            n154 = Merge Errors(w409) -> (w405:errorcluster)
          }
          frame "Exit" {
            w418 = 91  # 91: not all Exit messages will have an argument
            w422 = TRUE  # Stop the VI
            # "Release the message queue reference"
            # "#CodeNeeded - Add any required cleanup code here"
            # "Exit - Exit the application."
            n155 = Variant To Data(error in=w426, type=T3 {"Origin"="", "Module ID"=-1, "Exit via Stop Module Req?"=FALSE, "Wait for Module to stop?"=FALSE} ("Stop Argument"), Variant=w416) -> (data=w413:T3, error out=w417:errorcluster)
            n156 = call <vilib>:"Clear Errors.vi"("error in (no error)"=w417, "specific error code to clear (0: all)"=w418) -> ("error out"=w425:errorcluster)  [unwired: 4 in, 1 out]
            n157 = control-ref of="This VI"() -> (w411:refnum<vi>)
            n158 = call-dynamic "Delacor_lib_QMH_Release Message Queue.vi"("error in (no error)"=w425, "Message Queue"=w424) -> ("error out"=w421:errorcluster)  [unwired: 9 in]
            n159 = call "Handle Exit.vi"("Stop Argument"=w413, "Module Admin in"=w412, "VI reference"=w411) -> ("error out"=w419:errorcluster, "Wait for Stop?"=w414:bool)  [unwired: 7 in]
            n160 = Merge Errors(w419, w421) -> (w420:errorcluster)
          }
          frame Default {
            # "'Default' case only runs if there is a message that isn't defined in any of the other cases.  Output a programming error."
            n161 = property class="Mod Admin"(reference=w428) -> ("Accessors:Module ID"=w427:i32)  [unwired: 1 in, 2 out]
            n162 = call "Module Name--constant.vi"("Module ID"=w427) -> ("Module Name"=w429:string)  [unwired: 10 in]
            n163 = xnode "Error Ring"("parameter 0"=w430, "parameter 1"=w429) -> ("error out"=w431:errorcluster)
          }
        }
        n164 = call-dynamic "Delacor_lib_QMH_Error Handler - Message Handling Loop.vi"("error in (no error)"=w208, "Message Queue in"=w199) -> ("dup error in"=w198:errorcluster)  [unwired: 8 in, 1 out]
      }
    }
    frame Error {
      n165 = call "Synchronize Caller Events.vi"("Module Admin"=w443) -> ("Module Admin out"=w442:refnum<class "Delacor_lib_QMH_Cloneable Module Admin.lvclass">)  [unwired: 9 in, 1 out]
      n166 = property class="Mod Admin"(reference=w442) -> ("Accessors:Module ID"=w441:i32)  [unwired: 1 in, 2 out]
      n167 = call "Module Name--constant.vi"("Module ID"=w441) -> ("Module Name"=w446:string)  [unwired: 10 in]
      n168 = call "Remove.vi"("Module ID"=w441) -> ()  [unwired: 9 in, 2 out]
      n169 = Format Into String(format string="An error occurred during initialization. %s is no longer running.", w446) -> (resulting string=w444:string)  [unwired: 2 in, 1 out]
      n170 = call "Error Reported.vi"("Additional Information"=w444, "Error"=w447, "Module ID"=w441) -> ()  [unwired: 8 in, 1 out]
    }
  }
  n171 = Merge Errors(w15, w14) -> (w16:errorcluster)
  n172 = call "Close Module.vi"("error in (no error)"=w16, "Wait for stop?"=w4, "Module Admin in"=w6) -> ("error out"=w8:errorcluster, "External Launch"=w2:bool, "Module Admin out"=w5:refnum<class "Delacor_lib_QMH_Cloneable Module Admin.lvclass">)  [unwired: 6 in]
  n173 = Unregister For Events(event registration refnum=w12, error in=w8) -> (error out=w3:errorcluster)
  "error out" <- w3
  n174 = local write "Module Admin"(w5) -> ()
  n175 = case "External Launch?" shown="True" w2 {
    tunnel: w3 -> [_ w449]
    frame False {
    }
    frame True {
      n176 = case shown="No Error" w449 {
        frame No Error {
          n177 = invoke class="VI" method="FP.Close"() -> ()  [unwired: 3 in, 3 out]
        }
        frame Error {
          n178 = invoke class="VI" method="FP.Open"("Activate"=TRUE ("Activate?")) -> ()  [unwired: 4 in, 5 out]
        }
      }
    }
  }
